vi "CalibrateRawXYZ.vi"(9 "raw XYZ array":dbl[](array[numeric]), 10 "integration time":dbl, 11 "gain":dbl) -> (3 "XYZ array":dbl[](array[numeric]))   [LabVIEW 2011]
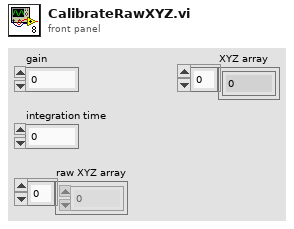
[diagram p1: front panel]
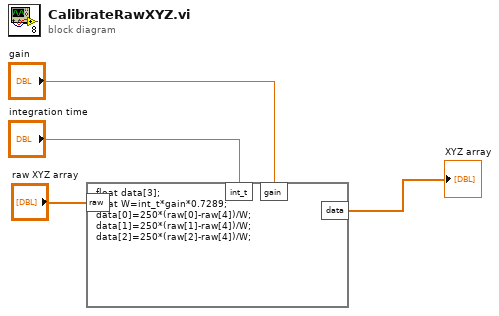
[diagram p0: block diagram]
diagram:
  n1 = formula code="float data[3]; \nfloat W=int_t*gain*0.7289;\ndata[0]=250*(raw[0]-raw[4])/W;\ndata[1]=250*(raw[1]-raw[4])/W;\ndata[2]=250*(raw[2]-raw[4])/W;"("raw"="raw XYZ array", "gain"="gain", "int_t"="integration time") -> ("data"=→"XYZ array":dbl[])
